vi "imageAverage.vi"(0 "Camera in":refnum<class "Camera.lvclass">, 5 "data_format":T2(ring)=enum."Mono16", 7 "crop":cluster{"x0":u64, "y0":u64, "x1":u64, "y1":u64}={"x0"=1, "y0"=1, "x1"=18446744073709551615, "y1"=18446744073709551615}, 11 "error in (no error)":errorcluster) -> (4 "Camera out":refnum<class "Camera.lvclass">, 6 "image (U8)":u8[][](array[numeric]), 8 "image (U32)":u32[][](array[numeric]), 10 "image (U64)":T1(array[cluster]), 13 "raw_image_8bit (U8)":u8[][](array[numeric]), 14 "raw_image (U16)":u16[][](array[numeric]), 15 "error out":errorcluster)   [LabVIEW 2019, in "Camera.lvclass"]
doc: "Get the averaged image. This image is calculated from all recorded images in the buffer.\nThe type of the image is 2D array of pixel values. This array is shaped depending on the resolution and ROI of the image. The data format determines which output is valid, but the raw_image(16) output is always valid.\n\nWe recommend that you do not use this function while recording is active, as it may give unexpected results. Typically you would record a number of images you want to average, then compute the average after all images have been recorded"
uses:
  Camera.lvclass
  Camera.lvclass/Camera.ctl
  pco.recorder/Recorder.lvlib
  pco.convert/Convert.lvlib
panel:
  out "rawFormat":enum16{"Word", "Byte"}(ring)
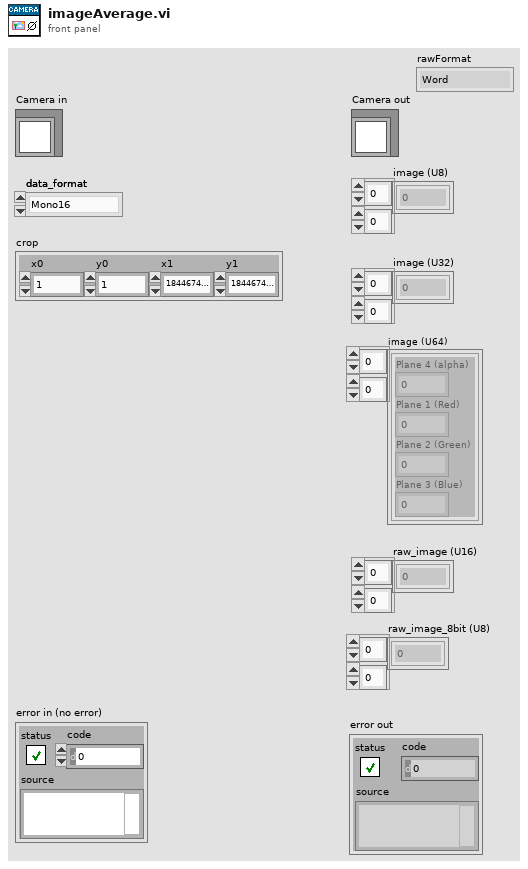
[diagram p1: front panel]
types:
  T1 = cluster{"Plane 4 (alpha)":u16, "Plane 1 (Red)":u16, "Plane 2 (Green)":u16, "Plane 3 (Blue)":u16}[][]
  T2 = enum16{"Undefined", "Mono8", "Mono16", "BGRA8", "RGBA8", "BGRA16", "RGBA16", "CompressedMono8"}
  T3 = map{enum16{"Undefined", "Mono8", "Mono16", "BGRA8", "RGBA8", "BGRA16", "RGBA16", "CompressedMono8"}, cluster{"sharpen":bool, "adaptive_sharpen":bool, "flip_vertical":bool, "auto_minmax":bool, "add_conv_flags":u32, "min_limit":u16, "max_limit":u16, "gamma":dbl, "contrast":i32, "pco_debayer_algorithm":bool, "color_temperature":i32, "color_saturation":i32, "color_vibrance":i32, "color_tint":i32, "lut_file":path}}
  T4 = map{enum16{"Undefined", "Mono8", "Mono16", "BGRA8", "RGBA8", "BGRA16", "RGBA16", "CompressedMono8"}, bool}
  T5 = cluster{"sharpen":bool, "adaptive_sharpen":bool, "flip_vertical":bool, "auto_minmax":bool, "add_conv_flags":u32, "min_limit":u16, "max_limit":u16, "gamma":dbl, "contrast":i32, "pco_debayer_algorithm":bool, "color_temperature":i32, "color_saturation":i32, "color_vibrance":i32, "color_tint":i32, "lut_file":path}
  T6 = map{enum16{"Undefined", "Mono8", "Mono16", "BGRA8", "RGBA8", "BGRA16", "RGBA16", "CompressedMono8"}, u64}
  T7 = cluster{"Blue":u16, "Green":u16, "Red":u16, "Alpha":u16}[][]
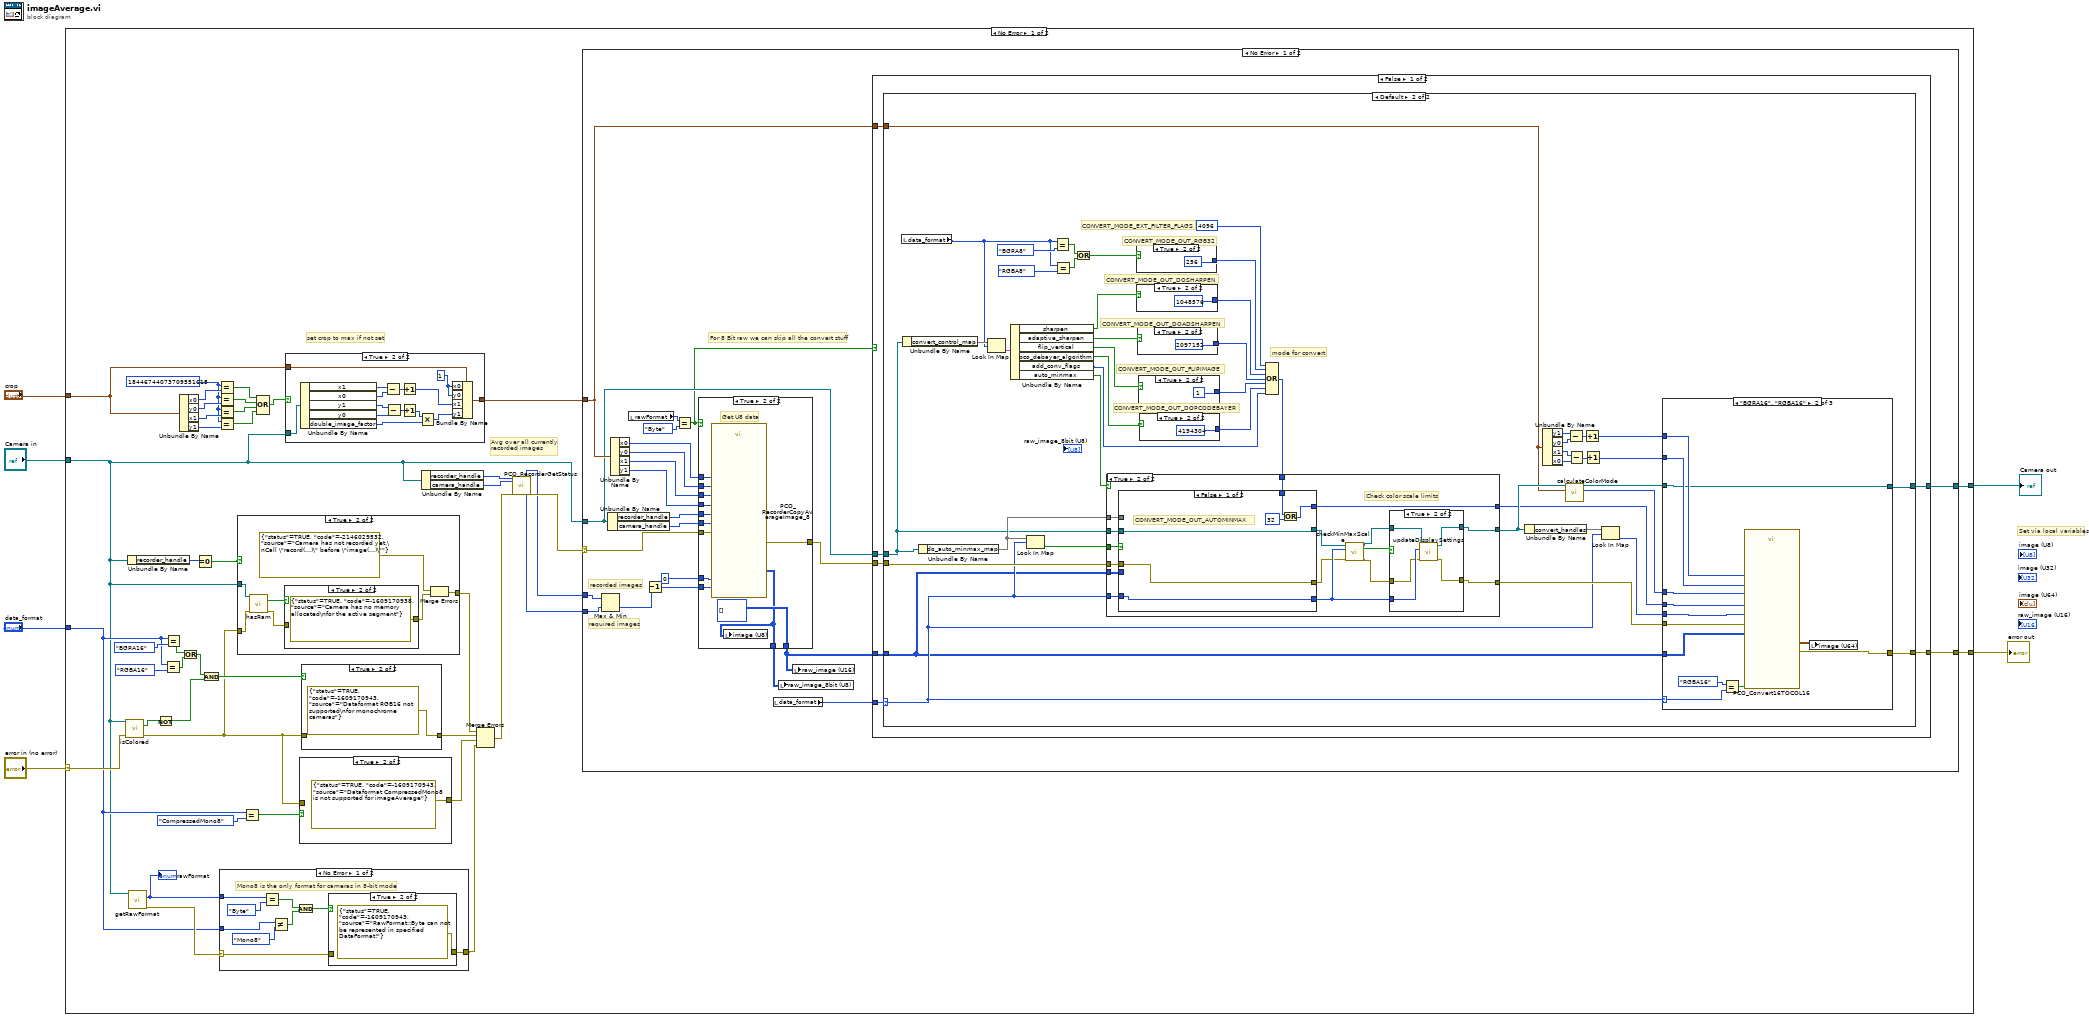
[diagram p0: block diagram]
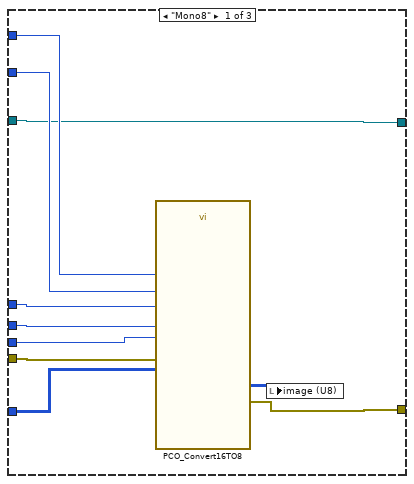
[diagram p7: hidden frame]
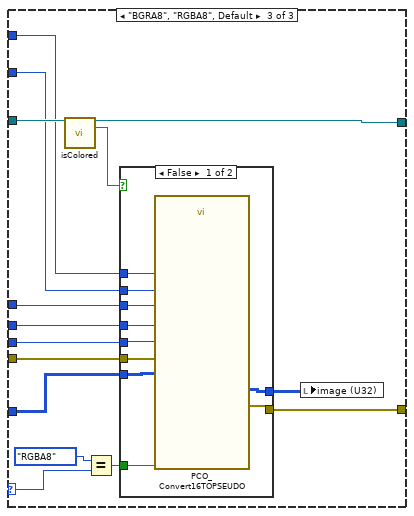
[diagram p8: hidden frame]
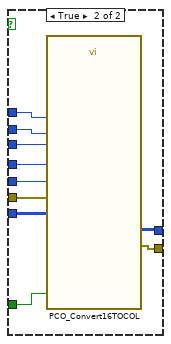
[diagram p9: hidden frame]
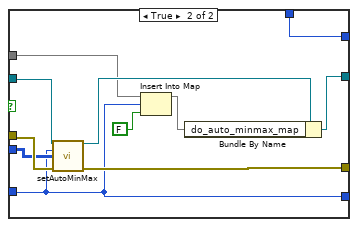
[diagram p12: hidden frame]
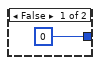
[diagram p13: hidden frame]
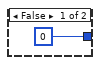
[diagram p14: hidden frame]
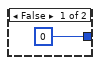
[diagram p15: hidden frame]
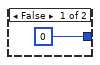
[diagram p16: hidden frame]
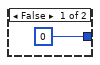
[diagram p17: hidden frame]
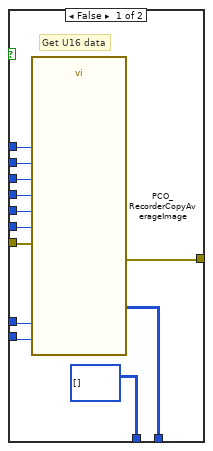
[diagram p19: hidden frame]
diagram:
  # "Set via local variables"
  n1 = case shown="No Error" "error in (no error)" {
    selector: "error in (no error)" -> [w22 w307]
    tunnel: [w29 w307] -> w3
    tunnel: [w30 w306] -> w2
    tunnel: "Camera in" -> [w8 w306]
    tunnel: "data_format" -> [w9 _]
    tunnel: "crop" -> [w32 _]
    frame No Error {
      w34 = u64 18446744073709551615 ("x0")
      # "Avg over all currently\nrecorded images"
      # "set crop to max if not set"
      n2 = call-dynamic "isColored.vi"("Camera in"=w8, "error in (no error)"=w22) -> ("colored"=w48:bool, "error out"=w13:errorcluster)  [unwired: 11 in, 1 out]
      n3 = Unbundle By Name(w8) -> ("recorder_handle"=w45:u64)
      n4 = call-dynamic "getRawFormat.vi"("Camera in"=w8) -> ("rawFormat"=w10:enum16{"Word", "Byte"}, "error out"=w11:errorcluster)  [unwired: 12 in, 1 out]
      "rawFormat" <- w10
      n5 = Not(x=w48) -> (.not. x?=w47:bool)
      n6 = Equal?(x=w9, y=T2."RGBA16" ("data_format")) -> (x = y?=w18:bool)
      n7 = Equal?(x=w9, y=T2."BGRA16" ("data_format")) -> (x = y?=w17:bool)
      n8 = Unbundle By Name(w32) -> ("x0"=w38:u64, "y0"=w37:u64, "x1"=w36:u64, "y1"=w35:u64)
      n9 = Or(x=w17, y=w18) -> (x .or. y?=w16:bool)
      n10 = Equal To 0?(x=w45) -> (x = 0?=w14:bool)
      n11 = And(x=w16, y=w47) -> (x .and. y?=w46:bool)
      n12 = Equal?(x=w34, y=w38) -> (x = y?=w39:bool)
      n13 = Equal?(x=w34, y=w37) -> (x = y?=w40:bool)
      n14 = Equal?(x=w34, y=w36) -> (x = y?=w41:bool)
      n15 = Equal?(x=w34, y=w35) -> (x = y?=w42:bool)
      n16 = case shown="No Error" w11 {
        selector: w11 -> [w50 w60]
        tunnel: w10 -> [w57 _]
        tunnel: w9 -> [w55 _]
        tunnel: [w49 w60] -> w7
        frame No Error {
          # "Mono8 is the only format for cameras in 8-bit mode"
          n17 = Equal?(x=w57, y=enum16{"Word", "Byte"}."Byte" ("rawFormat")) -> (x = y?=w53:bool)
          n18 = Not Equal?(x=w55, y=T2."Mono8" ("data_format")) -> (x != y?=w52:bool)
          n19 = And(x=w53, y=w52) -> (x .and. y?=w51:bool)
          n20 = case shown="True" w51 {
            tunnel: w50 -> [w58 _]
            tunnel: [w58 errorcluster {"status"=TRUE, "code"=-1609170943, "source"="RawFormat::Byte can not be represented in specified DataFormat!"} ("error constant")] -> w49
            frame False {
            }
            frame True {
            }
          }
        }
        frame Error {
        }
      }
      n21 = case shown="True" w14 {
        tunnel: w13 -> [w61 w67]
        tunnel: [w61 w62] -> w12
        tunnel: w8 -> [_ w68]
        frame False {
        }
        frame True {
          n22 = call-dynamic "hasRam.vi"("Camera in"=w68, "error in (no error)"=w67) -> ("hasRam"=w66:bool, "error out"=w65:errorcluster)  [unwired: 11 in, 1 out]
          n23 = case shown="True" w66 {
            tunnel: w65 -> [w69 _]
            tunnel: [w69 errorcluster {"status"=TRUE, "code"=-1609170938, "source"="Camera has no memory allocated\nfor the active segment"} ("error constant")] -> w63
            frame False {
            }
            frame True {
            }
          }
          n24 = Merge Errors(errorcluster {"status"=TRUE, "code"=-2146029532, "source"="Camera has not recorded yet.\nCall \"record(...)\" before \"image(...)\""} ("error constant"), w63) -> (w62:errorcluster)
        }
      }
      n25 = Equal?(x=w9, y=T2."CompressedMono8" ("data_format")) -> (x = y?=w21:bool)
      n26 = Compound Arithmetic op=OR(w39, w40, w41, w42) -> (w33:bool)
      n27 = case shown="True" w33 {
        tunnel: w8 -> [_ w301]
        tunnel: w32 -> [w287 w300]
        tunnel: [w287 w299] -> w31
        frame False {
        }
        frame True {
          w298 = u16 1 ("x0")
          n28 = Unbundle By Name(w301) -> ("x1"=w297:u64, "x0"=w296:u64, "y1"=w294:u64, "y0"=w293:u64, "double_image_factor"=w289:u16)
          n29 = Subtract(x=w297, y=w296) -> (x-y=w295:u64)
          n30 = Subtract(x=w294, y=w293) -> (x-y=w291:u64)
          n31 = Increment(x=w295) -> (x+1=w292:u64)
          n32 = Increment(x=w291) -> (x+1=w290:u64)
          n33 = Multiply(x=w290, y=w289) -> (x*y=w288:u64)
          n34 = Bundle By Name(cluster=w300, "x0"=w298, "y0"=w298, "x1"=w292, "y1"=w288) -> (w299:cluster{"x0":u64, "y0":u64, "x1":u64, "y1":u64})
        }
      }
      n35 = case shown="True" w21 {
        tunnel: [w304 errorcluster {"status"=TRUE, "code"=-1609170943, "source"="Dataformat CompressedMono8  is not supported for imageAverage"} ("error constant")] -> w43
        tunnel: w13 -> [w304 _]
        frame False {
        }
        frame True {
        }
      }
      n36 = case shown="True" w46 {
        tunnel: w13 -> [w302 _]
        tunnel: [w302 errorcluster {"status"=TRUE, "code"=-1609170943, "source"="Dataformat RGB16 not supported\nfor monochrome cameras"} ("error constant")] -> w44
        frame False {
        }
        frame True {
        }
      }
      n37 = Unbundle By Name(w8) -> ("recorder_handle"=w26:u64, "camera_handle"=w25:u64)
      n38 = Merge Errors(w12, w44, w43, w7) -> (w28:errorcluster)
      n39 = call "PCO_RecorderGetStatus.vi"("phRec"=w26, "phCam"=w25, "error in (no error)"=w28) -> ("dwProcImgCount"=w24:u32, "dwReqImgCount"=w23:u32, "error out"=w27:errorcluster)  [unwired: 5 in, 9 out]
      n40 = case shown="No Error" w27 {
        selector: w27 -> [w87 w286]
        tunnel: w31 -> [w84 _]
        tunnel: w8 -> [w80 w285]
        tunnel: [w83 w285] -> w30
        tunnel: [w82 w286] -> w29
        tunnel: w24 -> [w79 _]
        tunnel: w23 -> [w78 _]
        frame No Error {
          # "For 8 Bit raw we can skip all the convert stuff"
          # "required images"
          # "recorded images"
          n41 = Max & Min(x=w79, y=w78) -> (min(x,y)=w76:u32)  [unwired: 1 out]
          n42 = Unbundle By Name(w80) -> ("recorder_handle"=w92:u64, "camera_handle"=w93:u64)
          n43 = Unbundle By Name(w84) -> ("x0"=w88:u64, "y0"=w89:u64, "x1"=w90:u64, "y1"=w91:u64)
          n44 = local read "rawFormat"() -> (w75:enum16{"Word", "Byte"})
          n45 = Decrement(x=w76) -> (x-1=w77:u32)
          n46 = Equal?(x=w75, y=enum16{"Word", "Byte"}."Byte" ("rawFormat")) -> (x = y?=w71:bool)
          n47 = case shown="True" w71 {
            tunnel: w93 -> [w267 w284]
            tunnel: w92 -> [w268 w283]
            tunnel: w91 -> [w269 w282]
            tunnel: w90 -> [w270 w281]
            tunnel: w89 -> [w271 w280]
            tunnel: w88 -> [w272 w279]
            tunnel: w87 -> [w266 w278]
            tunnel: [w263 u16[][] []] -> w72
            tunnel: [w261 w277] -> w86
            tunnel: u32 0 ("dwStartIdx") -> [w265 w276]
            tunnel: w77 -> [w264 w275]
            tunnel: [u8[][] [] w273] -> w73
            frame False {
              # "Get U16 data"
              n48 = call "PCO_RecorderCopyAverageImage.vi"("phRec"=w268, "wRoiX0"=w272, "wRoiX1"=w270, "phCam"=w267, "dwStartIdx"=w265, "dwStopIdx"=w264, "error in (no error)"=w266, "wRoiY0"=w271, "wRoiY1"=w269) -> ("wImgBuf"=w263:u16[][], "error out"=w261:errorcluster)  [unwired: 3 in, 2 out]
            }
            frame True {
              # "Get U8 data"
              n49 = call "PCO_RecorderCopyAverageImage_8.vi"("phRec"=w283, "wRoiX0"=w279, "wRoiX1"=w281, "phCam"=w284, "dwStartIdx"=w276, "dwStopIdx"=w275, "error in (no error)"=w278, "wRoiY0"=w280, "wRoiY1"=w282) -> ("bImgBuf"=w273:u8[][], "error out"=w277:errorcluster)  [unwired: 3 in, 2 out]
              n50 = local write "image (U8)"(w273) -> ()
            }
          }
          n51 = local read "data_format"() -> (w85:T2)
          n52 = local write "raw_image_8bit (U8)"(w73) -> ()
          n53 = local write "raw_image (U16)"(w72) -> ()
          n54 = case shown="False" w71 {
            tunnel: w86 -> [w100 w259]
            tunnel: w85 -> [w99 _]
            tunnel: w84 -> [w98 _]
            tunnel: [w97 w260] -> w83
            tunnel: [w96 w259] -> w82
            tunnel: w80 -> [w95 w260]
            tunnel: w72 -> [w94 _]
            frame False {
              n55 = case shown="Default" w99 {
                selector: w99 -> [_ w115]
                tunnel: w100 -> [w101 w147]
                tunnel: w94 -> [_ w114]
                tunnel: w95 -> [w102 w126]
                tunnel: w98 -> [_ w144]
                tunnel: [w102 w111] -> w97
                tunnel: [w101 w112] -> w96
                frame "Mono16" {
                }
                frame Default {
                  # "CONVERT_MODE_OUT_RGB32"
                  # "CONVERT_MODE_OUT_FLIPIMAGE"
                  # "CONVERT_MODE_OUT_DOPCODEBAYER"
                  # "CONVERT_MODE_OUT_DOADSHARPEN"
                  # "CONVERT_MODE_OUT_DOSHARPEN"
                  # "CONVERT_MODE_EXT_FILTER_FLAGS"
                  # "mode for convert"
                  n56 = local read "data_format"() -> (w106:T2)
                  n57 = Unbundle By Name(w126) -> ("convert_control_map"=w125:T3)
                  n58 = Unbundle By Name(w126) -> ("do_auto_minmax_map"=w137:T4)
                  n59 = Look In Map(map=w125, key=w106) -> (value=w135:T5)  [unwired: 1 in, 1 out]
                  n60 = Unbundle By Name(w135) -> ("sharpen"=w134:bool, "adaptive_sharpen"=w133:bool, "flip_vertical"=w127:bool, "pco_debayer_algorithm"=w124:bool, "add_conv_flags"=w103:u32, "auto_minmax"=w104:bool)
                  n61 = Look In Map(map=w137, key=w115) -> (value=w136:bool)  [unwired: 1 in, 1 out]
                  n62 = Equal?(x=w106, y=T2."BGRA8" ("data_format")) -> (x = y?=w108:bool)
                  n63 = Equal?(x=w106, y=T2."RGBA8" ("data_format")) -> (x = y?=w107:bool)
                  n64 = Or(x=w108, y=w107) -> (x .or. y?=w105:bool)
                  n65 = case shown="True" w105 {
                    tunnel: [u32 0 ("image_index") u32 256 ("image_index")] -> w128
                    frame False {
                    }
                    frame True {
                    }
                  }
                  n66 = case shown="True" w134 {
                    tunnel: [u32 0 ("image_index") u32 1048576 ("image_index")] -> w132
                    frame False {
                    }
                    frame True {
                    }
                  }
                  n67 = case shown="True" w133 {
                    tunnel: [u32 0 ("image_index") u32 2097152 ("image_index")] -> w131
                    frame False {
                    }
                    frame True {
                    }
                  }
                  n68 = case shown="True" w127 {
                    tunnel: [u32 0 ("image_index") u32 1 ("image_index")] -> w130
                    frame False {
                    }
                    frame True {
                    }
                  }
                  n69 = case shown="True" w124 {
                    tunnel: [u32 0 ("image_index") u32 4194304 ("image_index")] -> w123
                    frame False {
                    }
                    frame True {
                    }
                  }
                  n70 = Compound Arithmetic op=OR(u32 4096 ("image_index"), w128, w132, w131, w130, w123, w103) -> (w122:u32)
                  n71 = case shown="True" w104 {
                    tunnel: w147 -> [w206 w224]
                    tunnel: [w207 w216] -> w145
                    tunnel: [w208 w223] -> w117
                    tunnel: w114 -> [_ w222]
                    tunnel: [w206 w215] -> w116
                    tunnel: w115 -> [_ w221]
                    tunnel: w137 -> [_ w220]
                    tunnel: w136 -> [_ w219]
                    tunnel: w126 -> [w207 w218]
                    tunnel: w122 -> [w208 w217]
                    frame False {
                    }
                    frame True {
                      # "Check color scale limits"
                      n72 = case shown="False" w219 {
                        tunnel: w218 -> [w234 w248]
                        tunnel: [w235 w240] -> w223
                        tunnel: w222 -> [_ w239]
                        tunnel: w221 -> [w232 w238]
                        tunnel: [w234 w246] -> w213
                        tunnel: w224 -> [w237 w245]
                        tunnel: [w237 w244] -> w212
                        tunnel: w220 -> [_ w243]
                        tunnel: w217 -> [w233 w240]
                        tunnel: [w232 w238] -> w214
                        frame False {
                          # "CONVERT_MODE_OUT_AUTOMINMAX"
                          n73 = Or(x=w233, y=u32 32 ("image_index")) -> (x .or. y?=w235:u32)
                        }
                        frame True {
                          n74 = call-dynamic "setAutoMinMax.vi"("Camera in"=w248, "data_format"=w238, "image"=w239, "error in (no error)"=w245) -> ("Camera out"=w247:refnum<class "Camera.lvclass">, "error out"=w244:errorcluster)  [unwired: 10 in]
                          n75 = Insert Into Map(map in=w243, key=w238, value=FALSE) -> (map out=w241:T4)  [unwired: 2 out]
                          n76 = Bundle By Name(cluster=w247, "do_auto_minmax_map"=w241) -> (w246:refnum<class "Camera.lvclass">)
                        }
                      }
                      n77 = call-dynamic "checkMinMaxScale.vi"("Camera in"=w213, "data_format"=w214, "error in (no error)"=w212) -> ("Camera out"=w211:refnum<class "Camera.lvclass">, "needsUpdate"=w209:bool, "error out"=w210:errorcluster)  [unwired: 10 in]
                      n78 = case shown="True" w209 {
                        tunnel: w211 -> [w226 w231]
                        tunnel: w210 -> [w225 w227]
                        tunnel: [w226 w229] -> w216
                        tunnel: [w225 w230] -> w215
                        tunnel: w214 -> [_ w228]
                        frame False {
                        }
                        frame True {
                          n79 = call-dynamic "updateDisplaySettings.vi"("Camera in"=w231, "data_format"=w228, "error in (no error)"=w227) -> ("Camera out"=w229:refnum<class "Camera.lvclass">, "error out"=w230:errorcluster)  [unwired: 11 in]
                        }
                      }
                    }
                  }
                  n80 = Unbundle By Name(w145) -> ("convert_handles"=w146:T6)
                  n81 = Unbundle By Name(w144) -> ("y1"=w142:u64, "y0"=w143:u64, "x1"=w141:u64, "x0"=w140:u64)
                  n82 = call-dynamic "calculateColorMode.vi"("Camera in"=w145, "crop"=w144) -> ("Camera out"=w119:refnum<class "Camera.lvclass">, "colorMode"=w118:i32)  [unwired: 11 in, 1 out]
                  n83 = Subtract(x=w142, y=w143) -> (x-y=w139:u64)
                  n84 = Subtract(x=w141, y=w140) -> (x-y=w138:u64)
                  n85 = Increment(x=w139) -> (x+1=w121:u64)
                  n86 = Increment(x=w138) -> (x+1=w120:u64)
                  n87 = Look In Map(map=w146, key=w115) -> (value=w113:u64)  [unwired: 1 in, 1 out]
                  n88 = case shown="\"BGRA16\", \"RGBA16\"" w115 {
                    selector: w115 -> [_ w160 w172]
                    tunnel: w113 -> [w152 w165 w178]
                    tunnel: w117 -> [w153 w166 w175]
                    tunnel: w118 -> [w154 w167 w174]
                    tunnel: w114 -> [w150 w168 w184]
                    tunnel: w121 -> [w156 w170 w177]
                    tunnel: w120 -> [w155 w169 w176]
                    tunnel: w116 -> [w151 w164 w179]
                    tunnel: w119 -> [w148 w162 w183]
                    tunnel: [w148 w162 w181] -> w111
                    tunnel: [w149 w163 w182] -> w112
                    frame "Mono8" {
                      n89 = call "PCO_Convert16TO8.vi"("ph"=w152, "height"=w156, "mode"=w153, "icolmode"=w154, "width"=w155, "error in (no error)"=w151, "b16"=w150) -> ("b8"=w157:u8[][], "error out"=w149:errorcluster)  [unwired: 5 in, 2 out]
                      n90 = local write "image (U8)"(w157) -> ()
                    }
                    frame "BGRA16", "RGBA16" {
                      n91 = Equal?(x=T2."RGBA16" ("data_format"), y=w160) -> (x = y?=w159:bool)
                      n92 = call "PCO_Convert16TOCOL16.vi"("ph"=w165, "height"=w170, "swap_colors"=w159, "mode"=w166, "icolmode"=w167, "width"=w169, "error in (no error)"=w164, "raw_image(U16)"=w168) -> ("image (U64)"=w158:T7, "error out"=w163:errorcluster)  [unwired: 4 in, 2 out]
                      n93 = local write "image (U64)"(w158) -> ()
                    }
                    frame "BGRA8", "RGBA8", Default {
                      n94 = call-dynamic "isColored.vi"("Camera in"=w183) -> ("Camera out"=w181:refnum<class "Camera.lvclass">, "colored"=w185:bool)  [unwired: 12 in, 1 out]
                      n95 = Equal?(x=T2."RGBA8" ("data_format"), y=w172) -> (x = y?=w171:bool)
                      n96 = case shown="False" w185 {
                        tunnel: w184 -> [w193 w203]
                        tunnel: [w195 w205] -> w182
                        tunnel: [w194 w204] -> w180
                        tunnel: w179 -> [w192 w202]
                        tunnel: w178 -> [w191 w201]
                        tunnel: w177 -> [w187 w200]
                        tunnel: w176 -> [w188 w199]
                        tunnel: w175 -> [w190 w198]
                        tunnel: w174 -> [w189 w197]
                        tunnel: w171 -> [w186 w196]
                        frame False {
                          n97 = call "PCO_Convert16TOPSEUDO.vi"("ph"=w191, "height"=w187, "swap_colors"=w186, "mode"=w190, "icolmode"=w189, "width"=w188, "error in (no error)"=w192, "b16"=w193) -> ("b32"=w194:u32[][], "error out"=w195:errorcluster)  [unwired: 4 in, 2 out]
                        }
                        frame True {
                          n98 = call "PCO_Convert16TOCOL.vi"("ph"=w201, "height"=w200, "swap_colors"=w196, "mode"=w198, "icolmode"=w197, "width"=w199, "error in (no error)"=w202, "b16"=w203) -> ("b32"=w204:u32[][], "error out"=w205:errorcluster)  [unwired: 4 in, 2 out]
                        }
                      }
                      n99 = local write "image (U32)"(w180) -> ()
                    }
                  }
                }
              }
            }
            frame True {
            }
          }
        }
        frame Error {
        }
      }
    }
    frame Error {
    }
  }
  "error out" <- w3
  "Camera out" <- w2
